vi "Write FP Refs.vi"(8 "error in (no error)":errorcluster, 10 "FP Refs":refnum<vi>[](array[refnum]), 11 "GUI Facade in":refnum<class "GUI Facade.lvclass">) -> (0 "error out":errorcluster, 3 "GUI Facade out":refnum<class "GUI Facade.lvclass">)   [LabVIEW 2018, in "GUI Facade.lvclass"]
uses:
  GUI Facade.lvclass
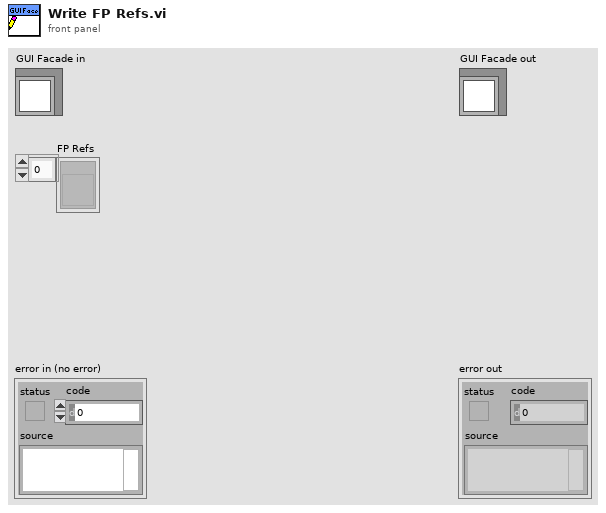
[diagram p1: front panel]
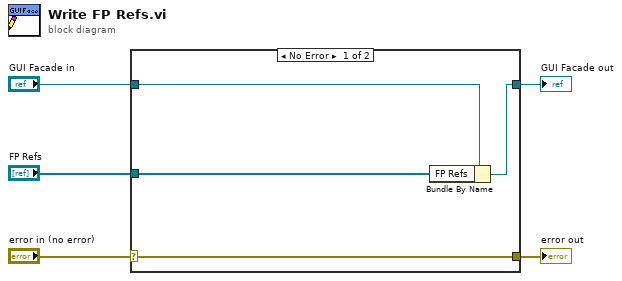
[diagram p0: block diagram]
diagram:
  n1 = case shown="No Error" "error in (no error)" {
    selector: "error in (no error)" -> [w9 w10]
    tunnel: [w9 w10] -> w4
    tunnel: [w7 w11] -> w2
    tunnel: "GUI Facade in" -> [w8 w11]
    tunnel: "FP Refs" -> [w6 _]
    frame No Error {
      n2 = Bundle By Name(cluster=w8, "FP Refs"=w6) -> (w7:refnum<class "GUI Facade.lvclass">)
    }
    frame Error {
    }
  }
  "error out" <- w4
  "GUI Facade out" <- w2
